vi "Offset Locking- Main v2.0.vi"() -> ()   [LabVIEW 2017]
uses:
  <vilib>/Utility/error.llb/DialogType.ctl
  <vilib>/measure/mamon.llb/Waveform Peak Detection for 1 Chan.vi
  <vilib>/addons/control/pid/pid.llb/PID Advanced (DBL).vi
  <vilib>/measure/NI_MAPro.lvlib
  <vilib>/addons/control/pid/NI_PID_pid.lvlib
  <vilib>/Analysis/NI_AALBase.lvlib
  <vilib>/measure/NI_MABase.lvlib
panel:
  in  "Minimum \namplitude\nfor peaks":dbl=0.5 format="%#_13g V"
  in  "PZT Voltage to \nFrequency Conversion":dbl format="%#_g V/GHz"
  out "PZT Chirp Output":waveform(dbl)(graph)
  in  "offset":dbl format="%0.2p V"
  in  "Sampling Info":cluster{"Fs":dbl, "#s":dbl}={"Fs"=1000.0, "#s"=1000.0} {"Fs" format="%.2p"}
  in  "frequency":dbl=1000.0 format="%0.2p Hz"
  in  "Chirp Amplitude":dbl=0.1 format="%0.2p GHz"
  in  "Run Chirp Program?":bool
  out "Run Time (min)":dbl
  out "standard deviation":dbl format="%0.3e"
  in  "Ref Peak 2":i32=1
  in  "Ref Peak":i32=2
  in  "First Cal Peak":i32
  in  "Last Cal Peak":i32=2
  out "# found":i32
  out "Offset":dbl(graph)
  in  "Manual PZT Control":dbl format="%#_g V"
  in  "Engage PZT PID?":bool
  out "Offset (GHz)":dbl format="%#_4g"
  in  "# of Shots for Averaging":i32=100
  in  "Name Convention":string="Chirp Offset Lock Log"
  in  "Save Directory":path=path "C:/Users/LabUser/Google Drive/Measurements/04-2018"
  out "Four peaks?":bool
  out "PZT Output":dbl(graph)
  in  "PID Gains":T1={"proportional gain (Kc)"=-1.0, "integral time (Ti, min)"=0.01, "derivative time (Td, min)"=0.0} {"derivative time (Td, min)" format="%.3f"; "integral time (Ti, min)" format="%.3f"; "proportional gain (Kc)" format="%.3f"}
  in  "Setpoint Range (GHz)":cluster{"setpoint high":dbl, "setpoint low":dbl}={"setpoint high"=7.7901, "setpoint low"=7.7899} {"setpoint high" format="%.4f"; "setpoint low" format="%.4f"}
  out "dt out (s)":dbl format="%.3f"
  in  "Frequency Offset Setpoint (GHz)":dbl=7.79 format="%.3f"
  out "GHz/sec":dbl
  out "dt":dbl format="%#_4g"
  out "Locations":dbl[](array[numeric]) format="%.2p"
  out "Amplitudes":dbl[](array[numeric]) format="%.2p"
  out "2nd Derivatives":dbl[](array[numeric]) format="%.2p"
  out "10 GHz FPI":dynamicdata(graph)
  in  "Stop":bool
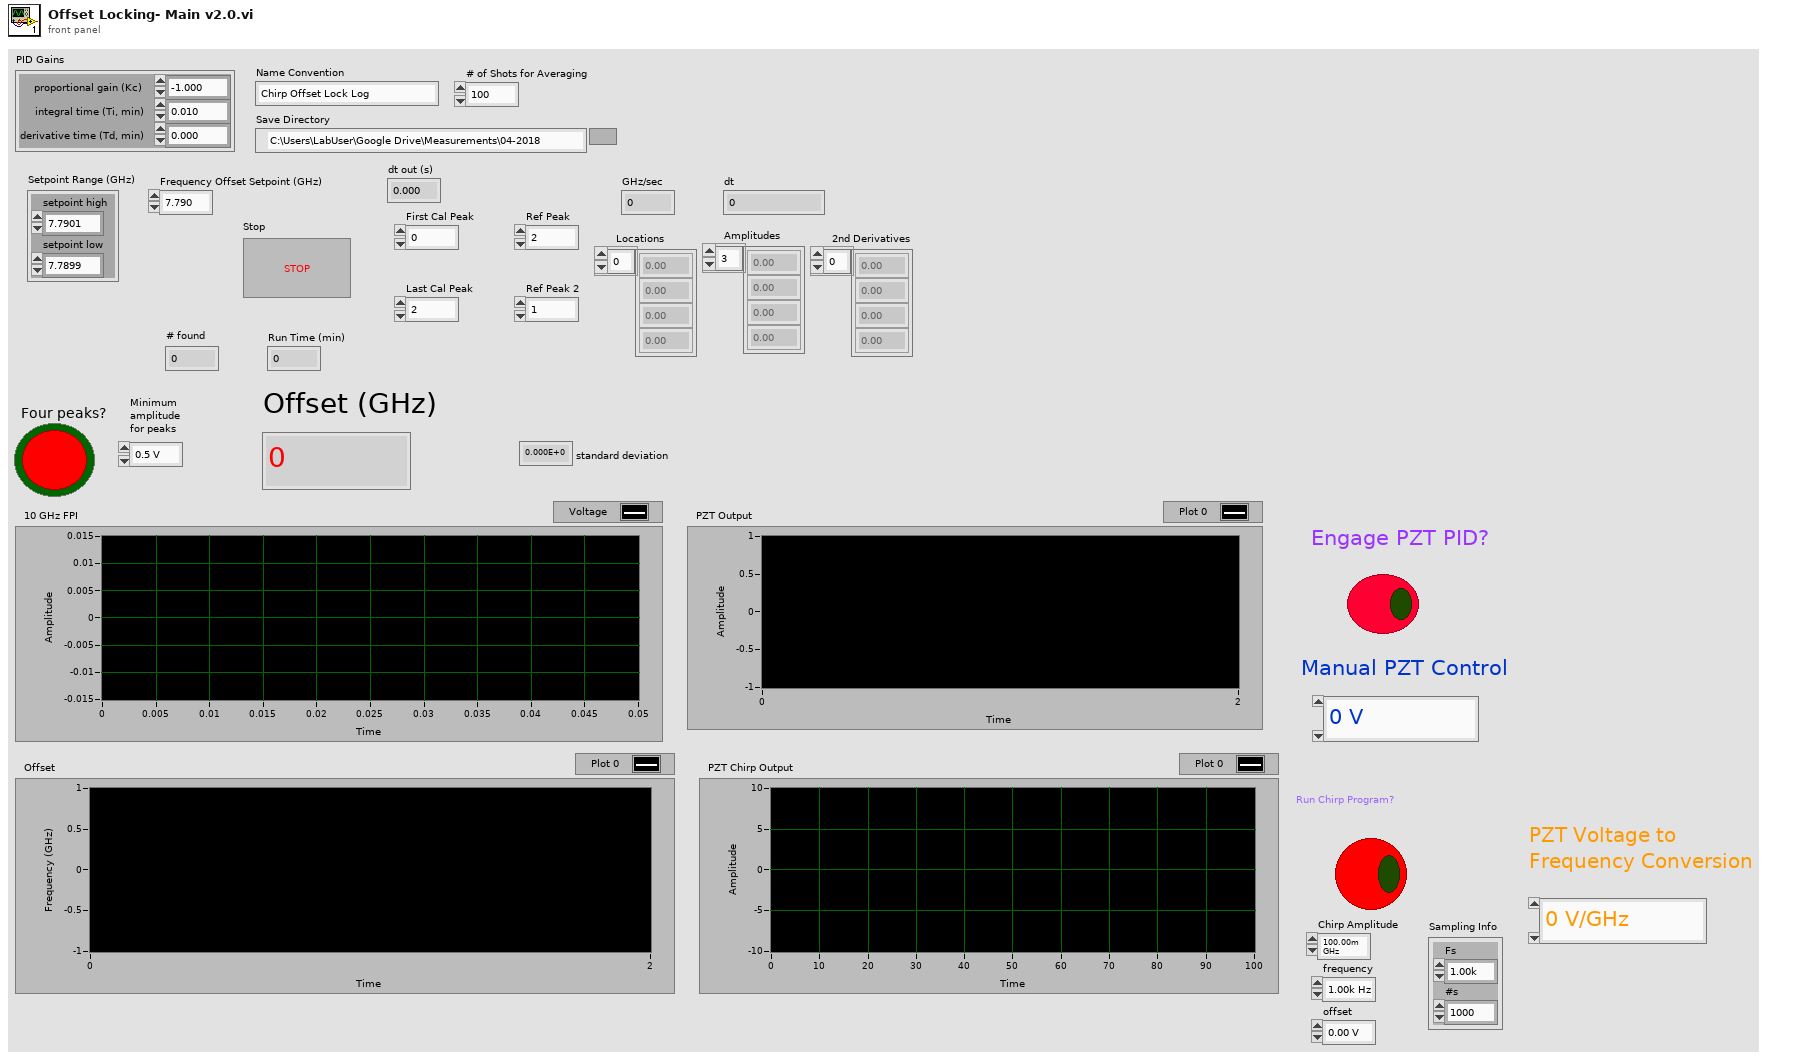
[diagram p1: front panel]
types:
  T1 = cluster{"proportional gain (Kc)":dbl, "integral time (Ti, min)":dbl, "derivative time (Td, min)":dbl}
  T2 = enum8{"Enabled", "Disabled", "Disabled and Grayed Out"}
  T3 = typedef "DialogType.ctl" = u16
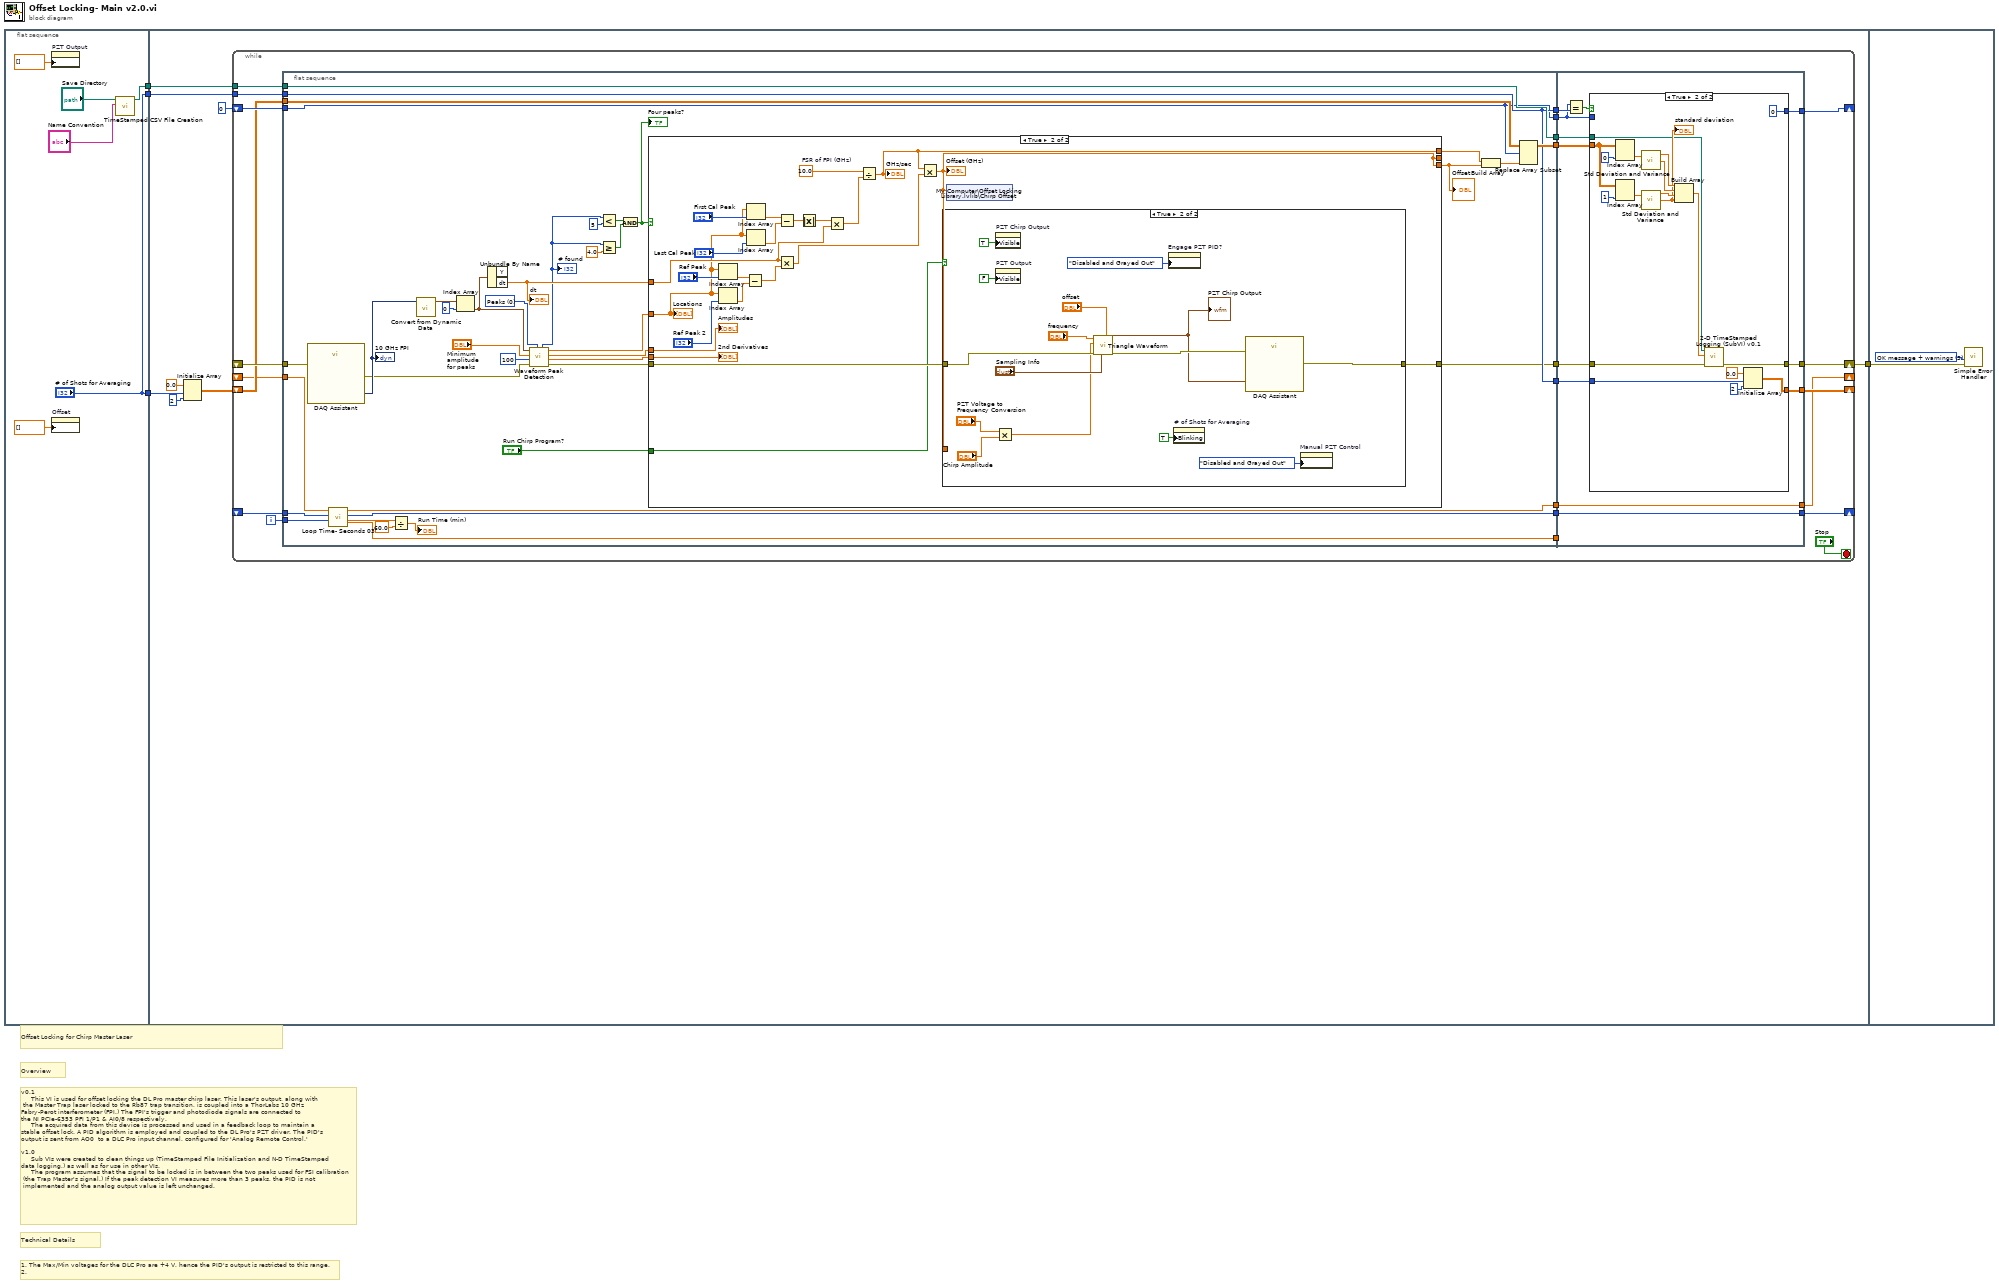
[diagram p0: block diagram]
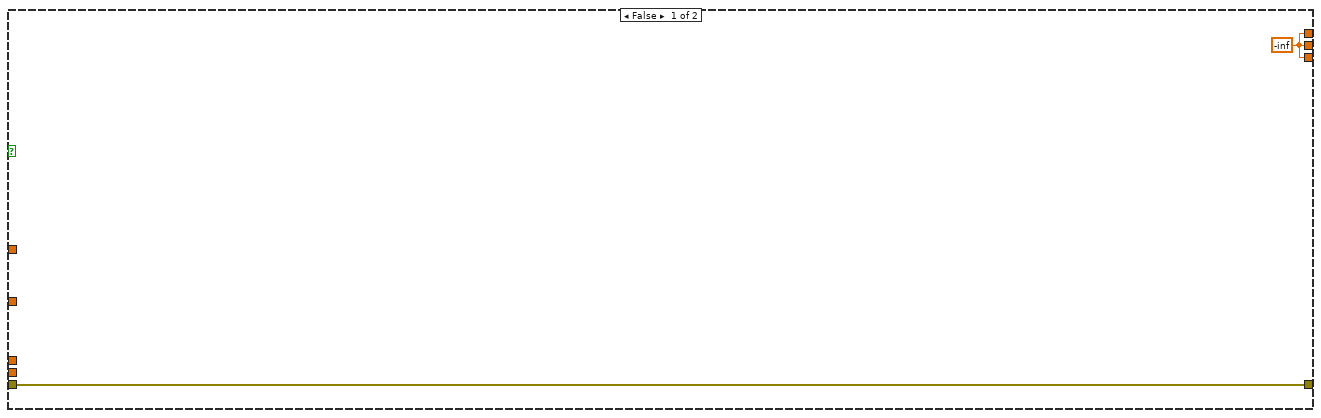
[diagram p2: hidden frame]
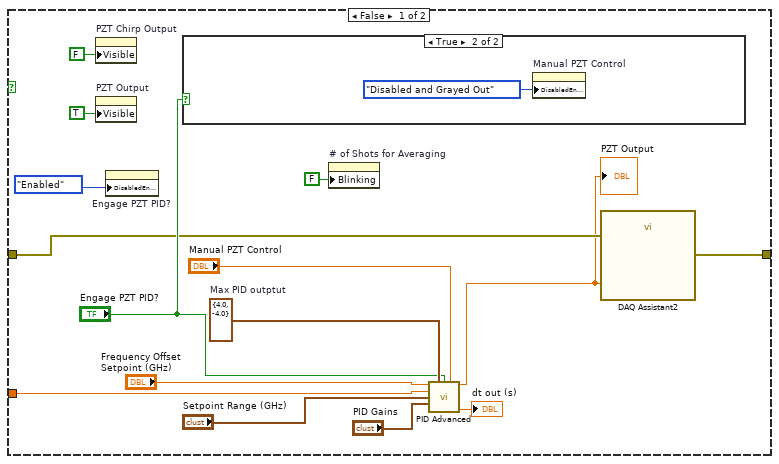
[diagram p3: hidden frame]
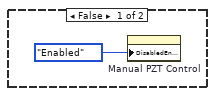
[diagram p4: hidden frame]
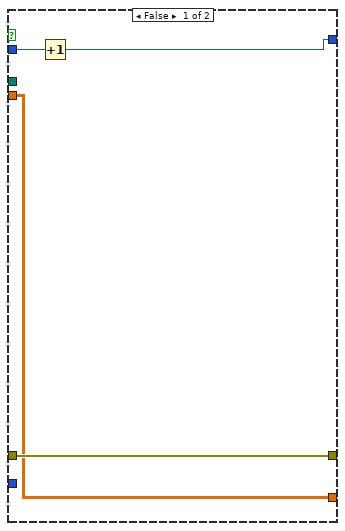
[diagram p5: hidden frame]
diagram:
  # "1. The Max/Min voltages for the DLC Pro are +4 V, hence the PID's output is restricted to this range.\n2."
  # "Technical Details"
  # "v0.1\n     This VI is used for offset locking the DL Pro master chirp laser. This laser's output, along with\n the Master Trap laser locked to the Rb87 trap transition, is coupled into a ThorLabs 10 GHz \nFabry-Perot interferometer (FPI.) The FPI's trigger and photodiode signals are connected to \nthe NI PCIe-6353 PFI 1/P1 & AI0/8 respectively. \n     The acquired data from this device is processed and used in a feedback loop to maintain a \nstable offset lock. A PID algorithm is employed and coupled to the DL Pro's PZT driver. The PID's\noutput is sent from AO0  to a DLC Pro input channel, configured for 'Analog Remote Control.'\n\nv1.0\n     Sub VIs were created to clean things up (TimeStamped File Initialization and N-D TimeStamped \ndata logging,) as well as for use in other VIs.\n     The program assumes that the signal to be locked is in between the two peaks used for FSI calibration\n (the Trap Master's signal.) If the peak detection VI measures more than 3 peaks, the PID is not\n implemented and the analog output value is left unchanged."
  # "Overview"
  # "Offset Locking for Chirp Master Laser"
  n1 = flat-sequence {
    tunnel: [w8] -> w4
    tunnel: ["# of Shots for Averaging"] -> w2
    tunnel: ["# of Shots for Averaging"] -> w1
    tunnel: w4 -> [w18]
    tunnel: [w17] -> w3
    tunnel: w2 -> [w15]
    tunnel: w1 -> [w12]
    tunnel: w3 -> [w171]
    frame #0 {
      n2 = property on="PZT Output" class="WFChart (strict)"("History Data"=dbl[] []) -> ()  [unwired: 2 in, 2 out]
      n3 = property on="Offset" class="WFChart (strict)"("History Data"=dbl[] []) -> ()  [unwired: 2 in, 2 out]
      n4 = call "TimeStamped CSV File Creation.vi"("Name Convention"="Name Convention", "Save Directory"="Save Directory") -> ("path"=w8:path)  [unwired: 8 in, 1 out]
    }
    frame #1 {
      n5 = Initialize Array(0.0 ("element"), w12, 2 ("dimension size")) -> (w14:dbl[][])
      n6 = while {
        shift-right: [w29] -> w17
        shift-left: _ -> [w40]
        tunnel: w18 -> [w38]
        shift-right: [w27] -> _
        shift-left: 0 -> [w36]
        tunnel: w15 -> [w34]
        shift-right: [w28] -> _
        shift-left: w14 -> [w31]
        shift-right: [w25] -> _
        shift-left: _ -> [w22]
        shift-right: [w23] -> _
        shift-left: _ -> [w21]
        i -> [w20]
        stop <- "Stop" stop-if-true
        n7 = flat-sequence {
          tunnel: w40 -> [w67]
          tunnel: [w43] -> w39
          tunnel: w38 -> [w65]
          tunnel: [w65] -> w37
          tunnel: w36 -> [w59]
          tunnel: [w59] -> w35
          tunnel: w34 -> [w60]
          tunnel: [w60] -> w33
          tunnel: [w64] -> w32
          tunnel: w31 -> [w63]
          tunnel: [w60] -> w30
          tunnel: [w58] -> w26
          tunnel: [w57] -> w24
          tunnel: w22 -> [w56]
          tunnel: w21 -> [w55]
          tunnel: w20 -> [w54]
          tunnel: [w46] -> w19
          tunnel: w39 -> [w142]
          tunnel: w37 -> [w143]
          tunnel: w35 -> [w140]
          tunnel: w33 -> [w148]
          tunnel: w32 -> [w145]
          tunnel: w30 -> [w146]
          tunnel: [w144] -> w29
          tunnel: [w141] -> w28
          tunnel: [w139] -> w27
          tunnel: w26 -> [w138]
          tunnel: [w138] -> w25
          tunnel: [w137] -> w23
          tunnel: w24 -> [w137]
          tunnel: w19 -> [_]
          frame #0 {
            w69 = u16 0 items=["Peaks", "Valleys"] ("peaks/valleys")
            n8 = call "DAQ Assistant"("error in"=w67) -> ("data"=w77:dynamicdata, "error out"=w66:errorcluster)  [unwired: 16 in, 1 out]
            "10 GHz FPI" <- w77
            n9 = call "Loop Time- Seconds 03.vi"("Loop Iteration"=w54, "Shift Registered Time In"=w55, "Shift Registered In"=w56) -> ("t"=w46:dbl, "Shift Registered Time Out"=w57:u32, "Shift Registered Out"=w58:dbl)  [unwired: 6 in]
            n10 = Divide(x=w46, y=60.0) -> (x/y=→"Run Time (min)":dbl)
            n11 = call "Convert from Dynamic Data"("Dynamic Data Type"=w77) -> ("Array of Waveform"=w79:waveform(dbl)[])  [unwired: 3 in]
            n12 = Index Array(array=w79, index=0) -> (element=w74:waveform(dbl))
            n13 = Unbundle By Name(w74) -> ("dt"=w72:dbl)  [unwired: 1 out]
            "dt" <- w72
            n14 = call-poly <vilib>:"Waveform Peak Detection.vi"("peaks/valleys"=w69, "error in"=w66, "width"=100, "threshold"="Minimum \namplitude\nfor peaks", "Signal In"=w74) -> ("error out"=w44:errorcluster, "2nd Derivatives"=w75:dbl[], "Amplitudes"=w76:dbl[], "Locations"=w73:dbl[], "# found"=w51:i32)  [unwired: 2 in]
            "# found" <- w51
            n15 = Less?(x=w51, y=5) -> (x < y?=w49:bool)
            n16 = Greater Or Equal?(x=w51, y=4.0) -> (x >= y?=w52:bool)
            n17 = And(x=w49, y=w52) -> (x .and. y?=w48:bool)
            "Four peaks?" <- w48
            n18 = case shown="True" w48 {
              tunnel: w76 -> [_ w104]
              tunnel: w75 -> [_ w103]
              tunnel: w73 -> [_ w87]
              tunnel: w72 -> [_ w94]
              tunnel: [w81 w92] -> w62
              tunnel: [w81 w85] -> w53
              tunnel: [w81 w85] -> _
              tunnel: w44 -> [w80 w84]
              tunnel: [w80 w83] -> w43
              tunnel: "Run Chirp Program?" -> [_ w82]
              frame False {
                w81 = -inf
              }
              frame True {
                w101 = 10.0  # FSR of FPI (GHz)
                n19 = Index Array(array=w87, index="Ref Peak") -> (element=w96:dbl)
                n20 = Index Array(array=w87, index="Ref Peak 2") -> (element=w86:dbl)
                n21 = Subtract(x=w96, y=w86) -> (x-y=w95:dbl)
                n22 = Index Array(array=w87, index="First Cal Peak") -> (element=w97:dbl)
                n23 = Index Array(array=w87, index="Last Cal Peak") -> (element=w102:dbl)
                n24 = Subtract(x=w97, y=w102) -> (x-y=w99:dbl)
                n25 = Multiply(x=w94, y=w95) -> (x*y=w93:dbl)
                n26 = Absolute Value(x=w99) -> (abs(x)=w98:dbl)
                n27 = Multiply(x=w98, y=w94) -> (x*y=w100:dbl)
                n28 = Divide(x=w101, y=w100) -> (x/y=w92:dbl)
                "GHz/sec" <- w92
                n29 = Multiply(x=w92, y=w93) -> (x*y=w85:dbl)
                "Offset (GHz)" <- w85
                n30 = case shown="True" w82 {
                  tunnel: w85 -> [w112 _]
                  tunnel: w84 -> [w111 w133]
                  tunnel: [w110 w131] -> w83
                  frame False {
                    w115 = cluster{"output high":dbl, "output low":dbl} {"output high"=4.0, "output low"=-4.0}  # Max PID outptut
                    n31 = property on="PZT Chirp Output" class="WFGraph (strict)"("Visible"=FALSE) -> ()  [unwired: 2 in, 2 out]
                    n32 = property on="PZT Output" class="WFChart (strict)"("Visible"=TRUE) -> ()  [unwired: 2 in, 2 out]
                    n33 = property on="Engage PZT PID?" class="Bool (strict)"("DisabledEnum"=T2."Enabled" ("Disabled")) -> ()  [unwired: 2 in, 2 out]
                    n34 = case shown="True" "Engage PZT PID?" {
                      frame False {
                        n35 = property on="Manual PZT Control" class="DigNum (strict)"("DisabledEnum"=T2."Enabled" ("Disabled")) -> ()  [unwired: 2 in, 2 out]
                      }
                      frame True {
                        n36 = property on="Manual PZT Control" class="DigNum (strict)"("DisabledEnum"=T2."Disabled and Grayed Out" ("Disabled")) -> ()  [unwired: 2 in, 2 out]
                      }
                    }
                    n37 = property on="# of Shots for Averaging" class="DigNum (strict)"("Blinking"=FALSE) -> ()  [unwired: 2 in, 2 out]
                    n38 = call-poly <vilib>:"PID Advanced.vi"("setpoint"="Frequency Offset Setpoint (GHz)", "output range"=w115, "auto? (T)"="Engage PZT PID?", "manual control"="Manual PZT Control", "process variable"=w112, "setpoint range"="Setpoint Range (GHz)", "PID gains"="PID Gains") -> ("output"=w109:dbl, "dt out (s)"=→"dt out (s)":dbl)  [unwired: 7 in]
                    "PZT Output" <- w109
                    n39 = call "DAQ Assistant2"("data"=w109, "error in"=w111) -> ("error out"=w110:errorcluster)  [unwired: 16 in, 1 out]
                  }
                  frame True {
                    n40 = property on="PZT Chirp Output" class="WFGraph (strict)"("Visible"=TRUE) -> ()  [unwired: 2 in, 2 out]
                    n41 = property on="PZT Output" class="WFChart (strict)"("Visible"=FALSE) -> ()  [unwired: 2 in, 2 out]
                    n42 = Multiply(x="PZT Voltage to \nFrequency Conversion", y="Chirp Amplitude") -> (x*y=w122:dbl)
                    n43 = call <vilib>:"Triangle Waveform.vi"("offset"="offset", "sampling info"="Sampling Info", "error in (no error)"=w133, "amplitude"=w122, "frequency"="frequency") -> ("error out"=w132:errorcluster, "signal out"=w129:waveform(dbl))  [unwired: 5 in]
                    "PZT Chirp Output" <- w129
                    n44 = property on="Engage PZT PID?" class="Bool (strict)"("DisabledEnum"=T2."Disabled and Grayed Out" ("Disabled")) -> ()  [unwired: 2 in, 2 out]
                    n45 = property on="# of Shots for Averaging" class="DigNum (strict)"("Blinking"=TRUE) -> ()  [unwired: 2 in, 2 out]
                    n46 = call "DAQ Assistant"("data"=w129, "error in"=w132) -> ("error out"=w131:errorcluster)  [unwired: 16 in, 1 out]
                    n47 = property on="Manual PZT Control" class="DigNum (strict)"("DisabledEnum"=T2."Disabled and Grayed Out" ("Disabled")) -> ()  [unwired: 2 in, 2 out]
                  }
                }
                n48 = shared-variable "My Computer\\Offset Locking Library.lvlib\\Chirp Offset"(w85) -> ()  [unwired: 1 in, 1 out]
                "2nd Derivatives" <- w103
                "Amplitudes" <- w104
                "Locations" <- w87
              }
            }
            "Offset" <- w53
            n49 = Build Array(w62, w53) -> (w61:dbl[])
            n50 = Replace Array Subset(array=w63, new element=w61, index (row)=w59) -> (w64:dbl[][])  [unwired: 1 in]
          }
          frame #1 {
            n51 = Equal?(x=w140, y=w148) -> (x = y?=w147:bool)
            n52 = case shown="True" w147 {
              tunnel: w146 -> [_ w155]
              tunnel: w145 -> [w151 w166]
              tunnel: [w152 w161] -> w144
              tunnel: w143 -> [_ w159]
              tunnel: w142 -> [w152 w158]
              tunnel: [w151 w154] -> w141
              tunnel: w140 -> [w150 _]
              tunnel: [w149 0] -> w139
              frame False {
                n53 = Increment(x=w150) -> (x+1=w149:i32)
              }
              frame True {
                n54 = Index Array(array=w166, index (col)=0 ("disabled index (col)")) -> (element=w169:dbl[])  [unwired: 1 in]
                n55 = Index Array(array=w166, index (col)=1 ("disabled index (col)")) -> (element=w167:dbl[])  [unwired: 1 in]
                n56 = call <vilib>:"Std Deviation and Variance.vi"("X"=w169) -> ("mean"=w165:dbl, "standard deviation"=w164:dbl)  [unwired: 1 in, 1 out]
                n57 = call <vilib>:"Std Deviation and Variance.vi"("X"=w167) -> ("mean"=w163:dbl, "standard deviation"=w162:dbl)  [unwired: 1 in, 1 out]
                "standard deviation" <- w162
                n58 = Build Array(w165, w164, w163, w162) -> (w160:dbl[])
                n59 = call "2-D TimeStamped Logging (SubVI) v0.1.vi"("error in (no error)"=w158, "array"=w160, "path"=w159) -> ("error out"=w161:errorcluster)  [unwired: 8 in]
                n60 = Initialize Array(0.0 ("element"), w155, 2 ("dimension size")) -> (w154:dbl[][])
              }
            }
          }
        }
      }
    }
    frame #2 {
      w172 = T3 3 items=["no dialog", "OK message", "continue or stop message", "OK message + warnings", "continue/stop + warnings"] ("type of dialog (OK msg:1)")
      n61 = call <vilib>:"Simple Error Handler.vi"("type of dialog (OK msg:1)"=w172, "error in (no error)"=w171) -> ()  [unwired: 3 in, 5 out]
    }
  }
